vi "Get Scanner Coarse.vi"(8 "error in (no error)":errorcluster, 11 "Translation Stages in":refnum<class "Translation Stages.lvclass">) -> (0 "error out":errorcluster, 2 "Default Scanner out":refnum<class "Scanner.lvclass">)   [LabVIEW 2015, in "Translation Stages.lvclass"]
doc: "(Dynamic) Returns the default Scanner object that scans over this Scannable. (Note that a Scannable may have multiple Scanners associated with it.) A Scanner is an analogue to an Iterator class in other languages."
uses:
  Translation Stages.lvclass
  Scanners/Scanner/Scanner.lvclass
  Scanners/Translation Stage Coarse/Translation Stage Coarse.lvclass
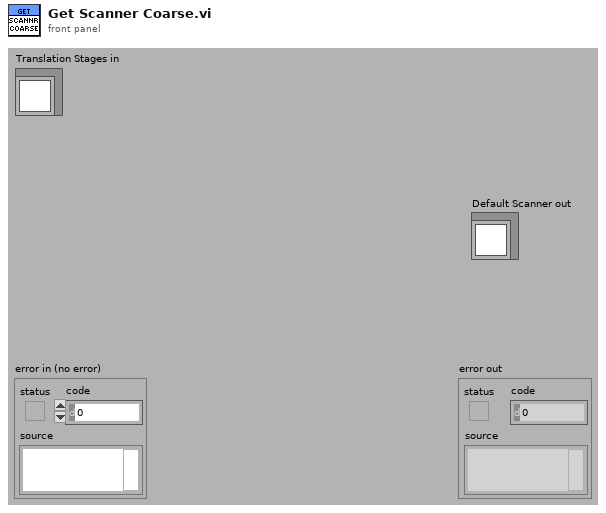
[diagram p1: front panel]
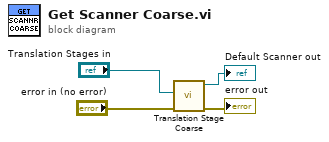
[diagram p0: block diagram]
diagram:
  n1 = call "Translation Stage Coarse.vi"("error in (no error)"="error in (no error)", "Translation Stages.lvclass"="Translation Stages in") -> ("error out"=→"error out":errorcluster, "Translation Stage Coarse Out"=→"Default Scanner out":refnum<class "Translation Stage Coarse.lvclass">)  [unwired: 8 in]
